vi "lv nominal create.vi"(8 "error in":errorcluster, 9 "base url":string="https://api.gov.nominal.io/api", 10 "workspace rid":string, 11 "api token":string) -> (0 "error out":errorcluster, 3 "client handle":i32)   [LabVIEW 2026]
uses:
  lv deref string.vi
  <vilib>/Utility/error.llb/Error Cluster From Error Code.vi
  bin/nominalClient_64.dll
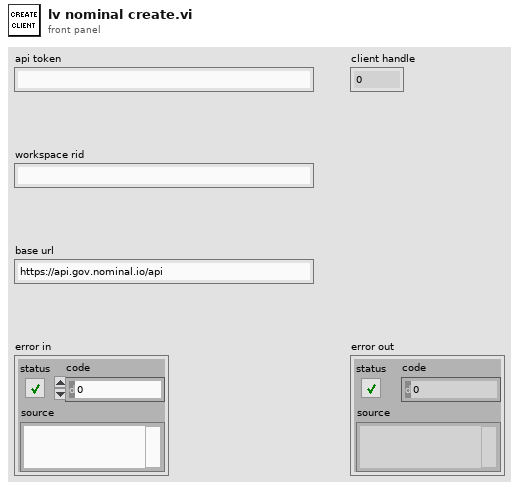
[diagram p1: front panel]
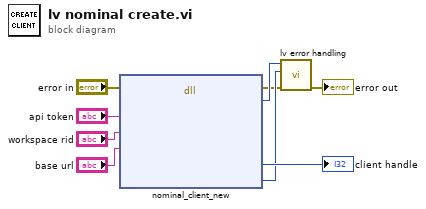
[diagram p0: block diagram]
diagram:
  n1 = dll-call lib="C:/sw/nominal-c/bin/nominalClient_64.dll" fn="nominal_client_new"(error in="error in", "api token"="api token", "workspace rid"="workspace rid", "base url"="base url") -> (error out=w2:errorcluster, "return type"=w3:i32, "client handle"=→"client handle":i32, "errorout"=w7:i32)  [unwired: 7 in, 1 out]
  n2 = call "lv error handling.vi"("error in"=w2, "error handle"=w7, "return code"=w3) -> ("error out"=→"error out":errorcluster)  [unwired: 8 in]
